vi "All Palette VIs.vi"   [LabVIEW 2020, in "NI_Data Type.lvlib"]
doc: "Contains all official, documented NI_Data Type.lvlib VIs."
uses:
  NI_Data Type.lvlib
  Data Type.ctl
types:
  T1 = typedef "NI_Data Type.lvlib/Data Type.ctl" = enum8{"Invalid Type", "Void", "I8", "I16", "I32", "I64", "U8", "U16", "U32", "U64", "Single Float", "Double Float", "Extended Float", "Single Complex", "Double Complex", "Extended Complex", "Enum U8", "Enum U16", "Enum U32", "Enum U64", "Single Float With Unit", "Double Float With Unit", "Extended Float With Unit", "Single Complex with Unit", "Double Complex with Unit", "Extended Complex with Unit", "Boolean", "String", "Path", "Picture", "Tag", "Array", "Cluster", "Variant", "LV Variant", "Waveform", "Timestamp", "Digital Waveform", "Digital Data", "ExpressData", "Refnum", "External Data", "VI", "Poly VI", "LabVIEW Class Instance", "Fixed Point", "Set Collection", "Map Collection"}
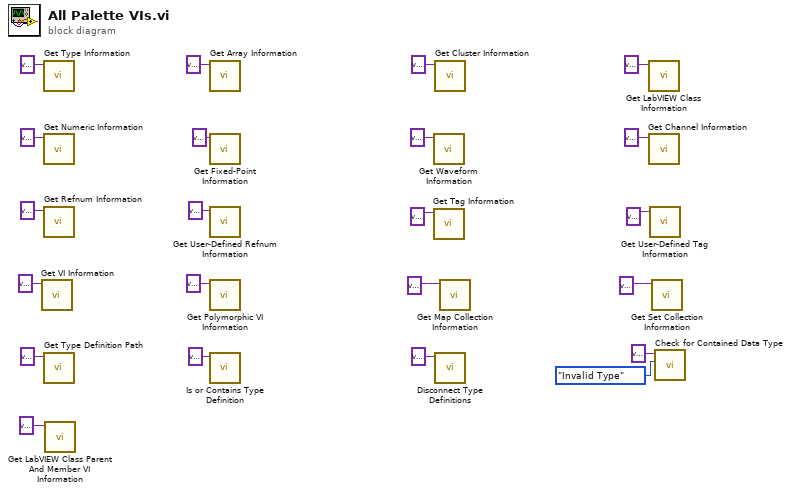
[diagram p0: block diagram]
diagram:
  n1 = call "Get VI Information.vi"("variant"=variant ("Variant")) -> ()  [unwired: 7 in, 4 out]
  n2 = call "Get Type Information.vi"("variant"=variant ("Variant")) -> ()  [unwired: 6 in, 5 out]
  n3 = call "Get Numeric Information.vi"("variant"=variant ("Variant")) -> ()  [unwired: 7 in, 4 out]
  n4 = call "Get Refnum Information.vi"("variant"=variant ("Variant")) -> ()  [unwired: 7 in, 4 out]
  n5 = call "Get Type Definition Path.vi"("variant"=variant ("Variant")) -> ()  [unwired: 9 in, 2 out]
  n6 = call "Get LabVIEW Class Parent And Member VI Information.vi"("variant"=variant ("Variant")) -> ()  [unwired: 7 in, 4 out]
  n7 = call "Get Array Information.vi"("variant"=variant ("Variant")) -> ()  [unwired: 7 in, 4 out]
  n8 = call "Get Fixed-Point Information.vi"("variant"=variant ("Variant")) -> ()  [unwired: 7 in, 4 out]
  n9 = call "Get User-Defined Refnum Information.vi"("variant"=variant ("Variant")) -> ()  [unwired: 7 in, 4 out]
  n10 = call "Get Polymorphic VI Information.vi"("variant"=variant ("Variant")) -> ()  [unwired: 9 in, 2 out]
  n11 = call "Is or Contains Type Definition.vi"("variant"=variant ("Variant")) -> ()  [unwired: 9 in, 2 out]
  n12 = call "Get Waveform Information.vi"("variant"=variant ("Variant")) -> ()  [unwired: 9 in, 2 out]
  n13 = call "Get Tag Information.vi"("variant"=variant ("Variant")) -> ()  [unwired: 9 in, 2 out]
  n14 = call "Get Cluster Information.vi"("variant"=variant ("Variant")) -> ()  [unwired: 9 in, 2 out]
  n15 = call "Disconnect Type Definitions.vi"("variant in"=variant ("Variant in")) -> ()  [unwired: 9 in, 2 out]
  n16 = call "Get Map Collection Information.vi"("variant"=variant ("Variant")) -> ()  [unwired: 8 in, 3 out]
  n17 = call "Get LabVIEW Class Information.vi"("variant"=variant ("Variant")) -> ()  [unwired: 8 in, 3 out]
  n18 = call "Get Channel Information.vi"("variant"=variant ("Variant")) -> ()  [unwired: 6 in, 5 out]
  n19 = call "Get User-Defined Tag Information.vi"("variant"=variant ("Variant")) -> ()  [unwired: 8 in, 3 out]
  n20 = call "Get Set Collection Information.vi"("variant"=variant ("Variant")) -> ()  [unwired: 9 in, 2 out]
  n21 = call "Check for Contained Data Type.vi"("data type to find"=Data_Type."Invalid Type" ("Data Type to Find"), "variant"=variant ("Variant")) -> ()  [unwired: 8 in, 2 out]
